vi "sub_DWA_dynamic-window.vi"(11 "x":dbl[](array[numeric])) -> (3 "dw":dbl[](array[numeric]))   [LabVIEW 2019]
uses:
  Ctrl/cmd_common.ctl
panel:
  out "Vd":dbl[](array[numeric])
  out "Vs":dbl[](array[numeric])
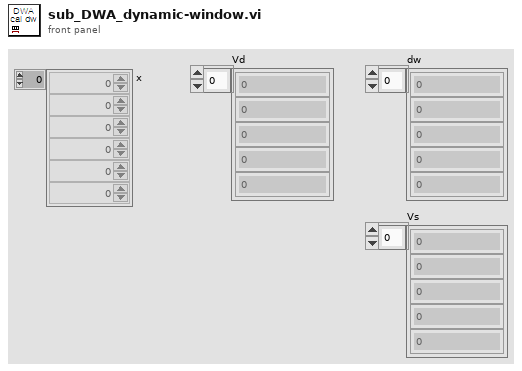
[diagram p1: front panel]
types:
  T1 = typedef "cmd_common.ctl" = enum16{"read", "write"}
  T2 = cluster{"max speed":dbl, "min speed":dbl, "max yaw rate":dbl, "max accel":dbl, "max delta yaw rate":dbl, "v resolution":dbl, "yaw rate resolution":dbl, "dt":dbl, "predict time":dbl, "to goal cost gain":dbl, "speed cost gain":dbl, "obstacle cost gain":dbl, "robot stuck flag cons":dbl, "robot type":enum16{"circle", "rectangle"}, "robot radius":dbl, "robot width":dbl, "robot length":dbl, "obstacles":cluster{"x":dbl, "y":dbl}[], "goal pt":cluster{"x":i32, "y":i32}}
  T3 = cluster{"x":dbl[], "dw":dbl[], "u":cluster{"v":dbl, "y":dbl}, "trajectory":dbl[][], "best trajectory":dbl[][], "best u":cluster{"v":dbl, "y":dbl}}
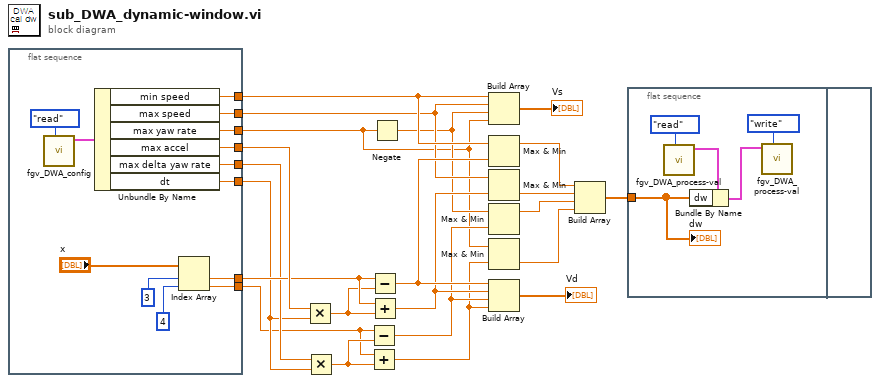
[diagram p0: block diagram]
diagram:
  n1 = flat-sequence {
    tunnel: [w31] -> w21
    tunnel: [w30] -> w20
    tunnel: [w29] -> w17
    tunnel: [w28] -> w16
    tunnel: [w27] -> w15
    tunnel: [w26] -> w13
    tunnel: [w25] -> w11
    tunnel: [w24] -> w7
    frame #0 {
      n2 = call "fgv_DWA_config.vi"("cmd"=cmd_common."read") -> ("config out"=w34:T2)  [unwired: 10 in]
      n3 = Unbundle By Name(w34) -> ("min speed"=w26:dbl, "max speed"=w25:dbl, "max yaw rate"=w24:dbl, "max accel"=w31:dbl, "max delta yaw rate"=w29:dbl, "dt"=w28:dbl)
      n4 = Index Array(array="x", index #1=3 ("index"), index #2=4 ("index")) -> (element #1=w30:dbl, element #2=w27:dbl)
    }
  }
  n5 = Multiply(x=w21, y=w16) -> (x*y=w19:dbl)
  n6 = Multiply(x=w17, y=w16) -> (x*y=w18:dbl)
  n7 = Subtract(x=w15, y=w18) -> (x-y=w8:dbl)
  n8 = Add(x=w15, y=w18) -> (x+y=w6:dbl)
  n9 = Subtract(x=w20, y=w19) -> (x-y=w12:dbl)
  n10 = Add(x=w20, y=w19) -> (x+y=w10:dbl)
  n11 = Negate(x=w7) -> (-x=w9:dbl)
  n12 = Build Array(w13, w11, w9, w7) -> (→"Vs":dbl[])
  n13 = Max & Min(x=w13, y=w12) -> (max(x,y)=w5:dbl)  [unwired: 1 out]
  n14 = Max & Min(x=w11, y=w10) -> (min(x,y)=w4:dbl)  [unwired: 1 out]
  n15 = Max & Min(x=w9, y=w8) -> (max(x,y)=w3:dbl)  [unwired: 1 out]
  n16 = Max & Min(x=w7, y=w6) -> (min(x,y)=w2:dbl)  [unwired: 1 out]
  n17 = Build Array(w12, w10, w8, w6) -> (→"Vd":dbl[])
  n18 = Build Array(w5, w4, w3, w2) -> (w1:dbl[])
  n19 = flat-sequence {
    tunnel: w1 -> [w36]
    frame #0 {
      n20 = call "fgv_DWA_process-val.vi"("cmd"=cmd_common."read") -> ("prcess val out"=w38:T3)  [unwired: 10 in]
      n21 = Bundle By Name(cluster=w38, "dw"=w36) -> (w37:T3)
      n22 = call "fgv_DWA_process-val.vi"("cmd"=cmd_common."write", "prcess val"=w37) -> ()  [unwired: 9 in, 1 out]
      "dw" <- w36
    }
    frame #1 {
    }
  }
